vi "Evaluate Polynomial with Matrix.vi"   [LabVIEW 2020, in "NI_AALPro.lvlib"]
doc: "Evaluates the polynomial <B>P(x)</B> with matrix <B>A</B>. The data types you wire to the <B>P(x)</B> and <B>A</B> inputs determine the polymorphic instance to use."
uses:
  NI_AALPro.lvlib
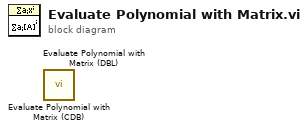
[diagram p0: block diagram]
diagram:
  n1 = call "Evaluate Polynomial with Matrix (CDB).vi"() -> ()  [unwired: 2 in, 2 out]
  n2 = call "Evaluate Polynomial with Matrix (DBL).vi"() -> ()  [unwired: 2 in, 2 out]
